vi "WSVCAP SHL Host LL Core.vi"(0 "Message In":string, 11 "error in":errorcluster, 12 "Log (T)":bool=TRUE, 13 "Function":T3) -> (3 "System":T1={"Settings"={"FPGA Resource Name"="", "I2C Slave Address"=20, "I2C Clock Rate (Hz)"=50000.0, "SPI Clock Rate (Hz)"=50000.0, "RFFE Slave Address"=20, "RFFE Clock Rate (Hz)"=50000.0, "Simulate FPGA"=TRUE, "C1 Cap DAC Default"=165, "C2 Cap DAC Default"=134, "C3 Cap DAC Default"=150}, "FPGA Resource"="", "Online"=FALSE, "I2C Wait Ticks"=0, "SPI Wait Ticks"=0, "RFFE Wait Ticks"=0} {"Settings"."C3 Cap DAC Default" format="0x%02x"; "Settings"."C2 Cap DAC Default" format="0x%02x"; "Settings"."C1 Cap DAC Default" format="0x%02x"; "Settings"."RFFE Clock Rate (Hz)" format="%.0f Hz"; "Settings"."RFFE Slave Address" format="0x%02x"; "Settings"."I2C Clock Rate (Hz)" format="%.0f Hz"; "Settings"."SPI Clock Rate (Hz)" format="%.0f Hz"; "Settings"."I2C Slave Address" format="0x%02x"}, 4 "Message Out":string, 15 "error out":errorcluster)   [LabVIEW 2012]
uses:
  Type Defs/WSVCAP SHL Function Enum.ctl
  Type Defs/WSVCAP SHL Core System Cluster.ctl
  Type Defs/WSVCAP SHL I2C Settings Cluster.ctl
  user.lib/Utilities/Type Defs/MISC IO Choice Enum.ctl
  Type Defs/WSVCAP SHL Top Level Control Operation Enum.ctl
  Type Defs/WSVCAP SHL Top Level Control Enum.ctl
  Type Defs/WSVCAP SHL Manager Operation Enum.ctl
  user.lib/Configuration Files/Type Defs/CFG File Operation Enum.ctl
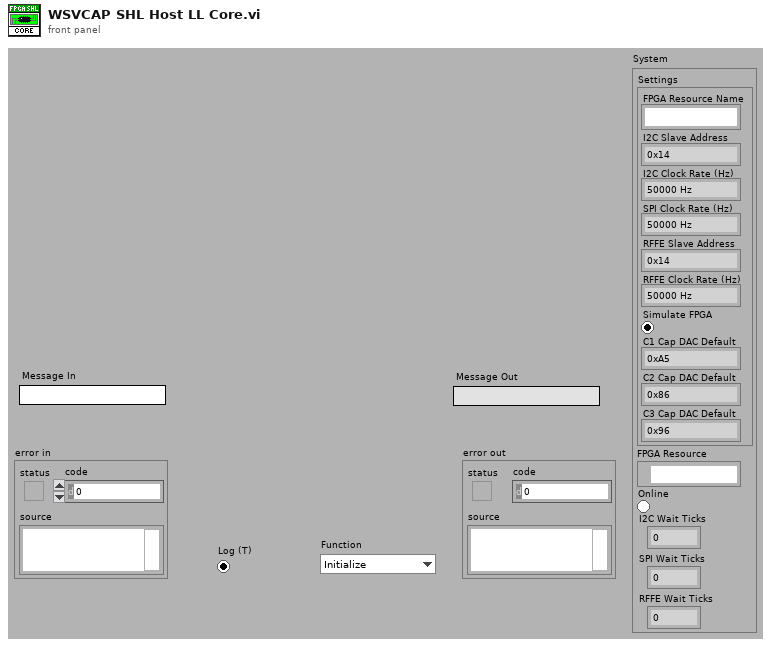
[diagram p1: front panel]
types:
  T1 = typedef "WSVCAP SHL Core System Cluster.ctl" = cluster{"Settings":T2, "FPGA Resource":tag, "Online":bool, "I2C Wait Ticks":u32, "SPI Wait Ticks":u32, "RFFE Wait Ticks":u32}
  T2 = typedef "WSVCAP SHL I2C Settings Cluster.ctl" = cluster{"FPGA Resource Name":string, "I2C Slave Address":u8, "I2C Clock Rate (Hz)":dbl, "SPI Clock Rate (Hz)":dbl, "RFFE Slave Address":u8, "RFFE Clock Rate (Hz)":dbl, "Simulate FPGA":bool, "C1 Cap DAC Default":u8, "C2 Cap DAC Default":u8, "C3 Cap DAC Default":u8}
  T3 = typedef "WSVCAP SHL Function Enum.ctl" = enum16{"Initialize", "Configure I2C", "Configure SPI", "Configure RFFE", "Write I2C", "Read I2C", "Write/Read SPI", "Start SPI Cycle", "Stop SPI Cycle", "Write RFFE", "Read RFFE", "Start RFFE Cycle", "Stop RFFE Cycle", "Get Status", "Close"}
  T4 = typedef "MISC IO Choice Enum.ctl" = enum16{"Read", "Write"}
  T5 = typedef "CFG File Operation Enum.ctl" = enum16{"Read", "Write", "Copy", "Edit"}
  T6 = typedef "WSVCAP SHL Manager Operation Enum.ctl" = enum16{"Initialize", "Close"}
  T7 = typedef "WSVCAP SHL Top Level Control Enum.ctl" = enum16{"Start", "Cmd", "Transaction", "Wait Ticks", "Socket Mask", "Slave Address", "Sub Address", "Bytes to Write", "Bytes to Read", "Write Data", "Write Flag", "Read Data", "Read Flag", "Ack Read", "Read Status Flag", "Ack Read Status", "Status", "Cycle Count", "Stop Cycle", "Exit"}
  T8 = typedef "WSVCAP SHL Top Level Control Operation Enum.ctl" = enum16{"Initialize", "Set Control", "Read Control", "Close"}
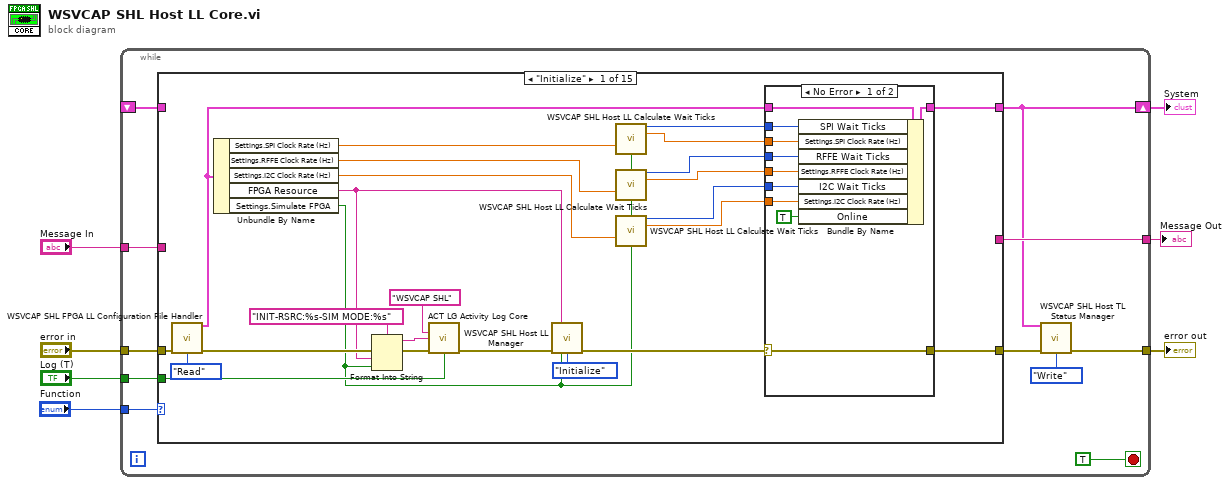
[diagram p0: block diagram]
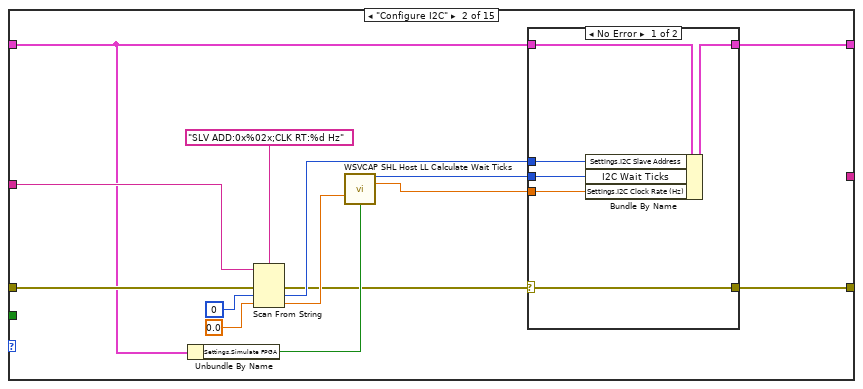
[diagram p3: hidden frame]
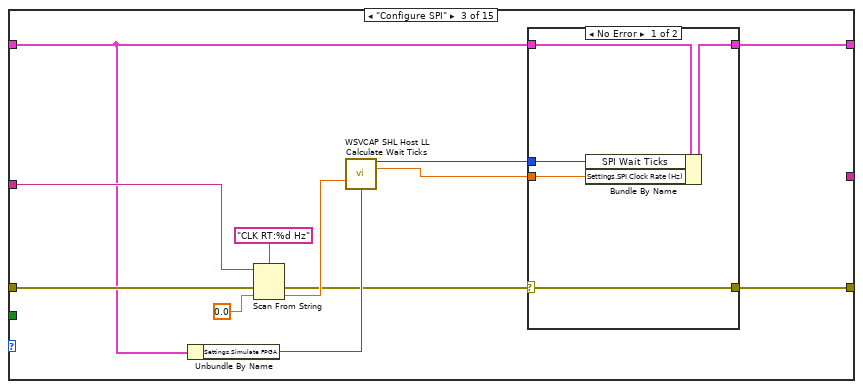
[diagram p5: hidden frame]
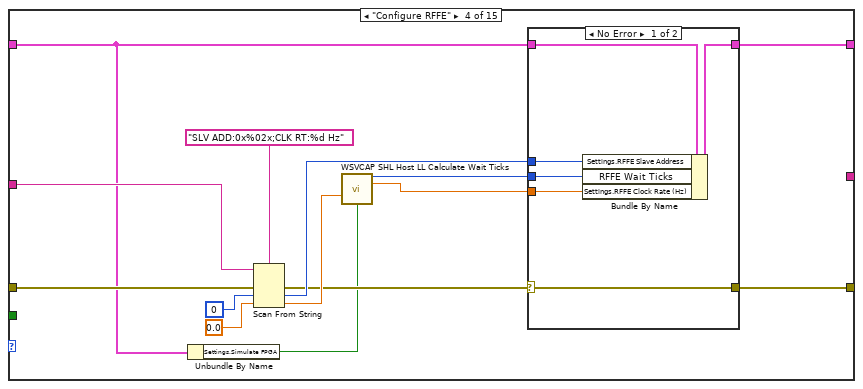
[diagram p7: hidden frame]
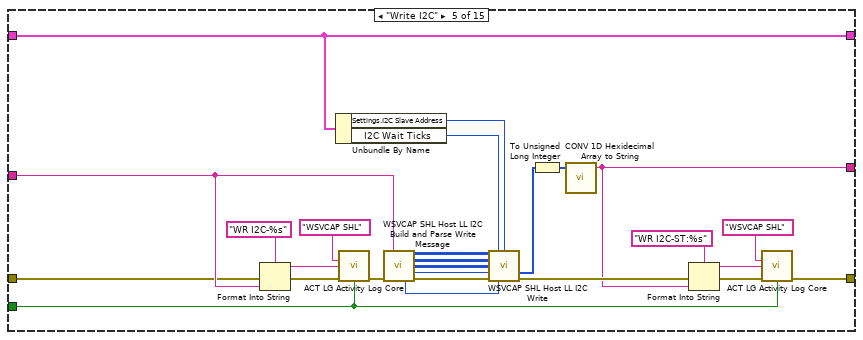
[diagram p9: hidden frame]
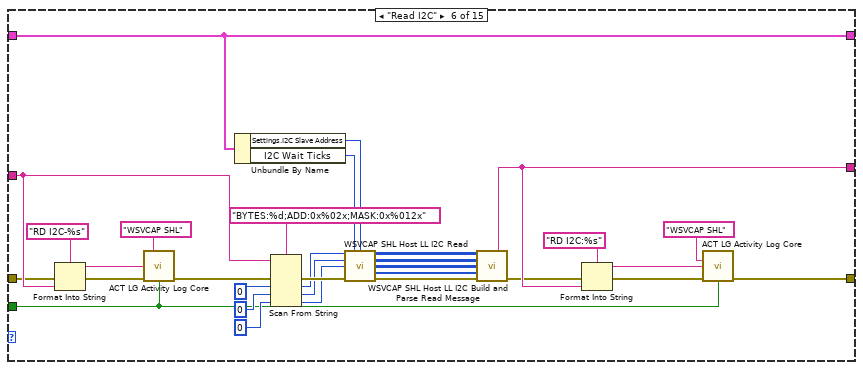
[diagram p10: hidden frame]
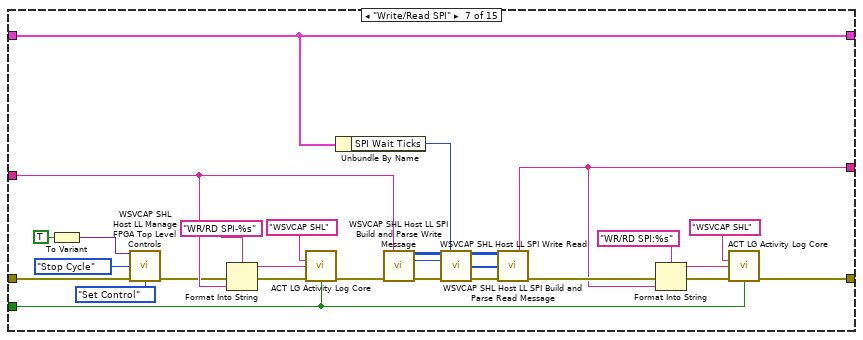
[diagram p11: hidden frame]
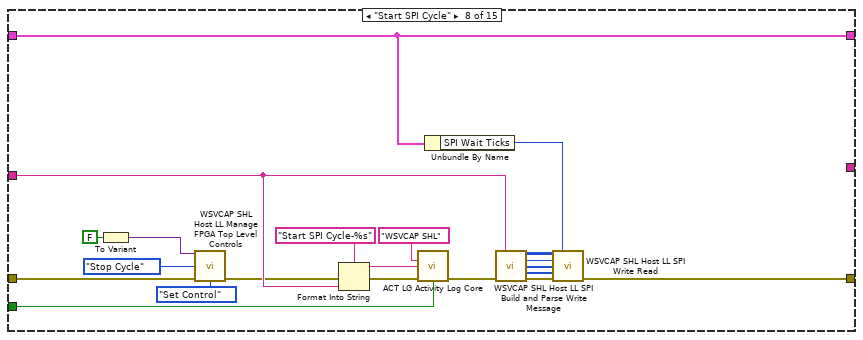
[diagram p12: hidden frame]
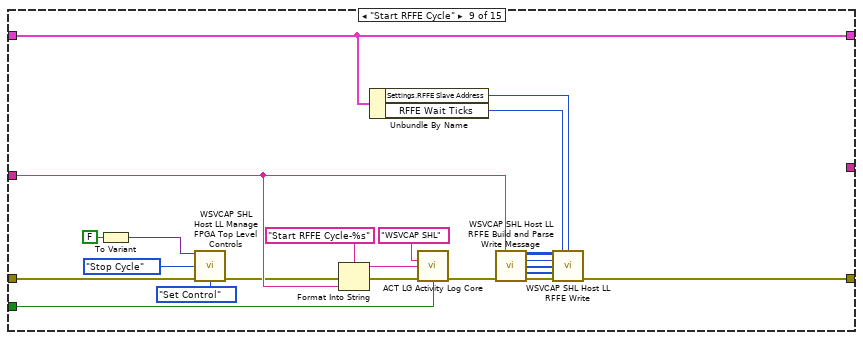
[diagram p13: hidden frame]
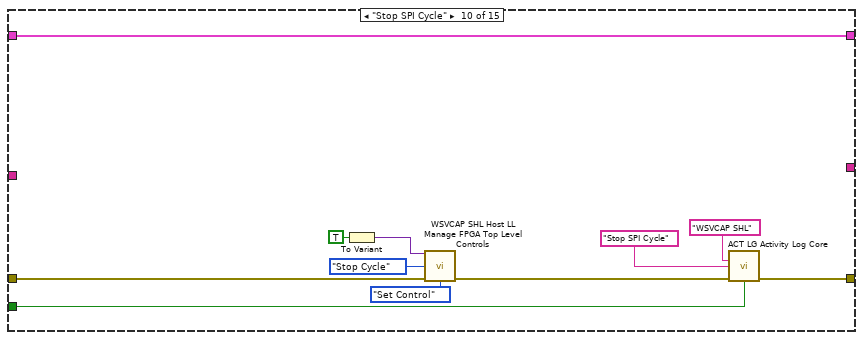
[diagram p14: hidden frame]
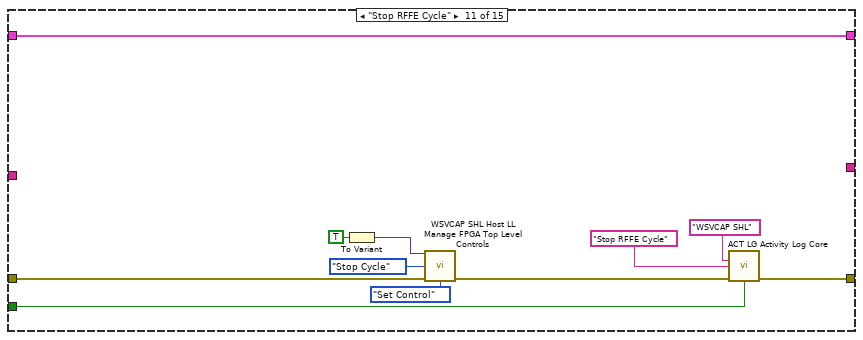
[diagram p15: hidden frame]
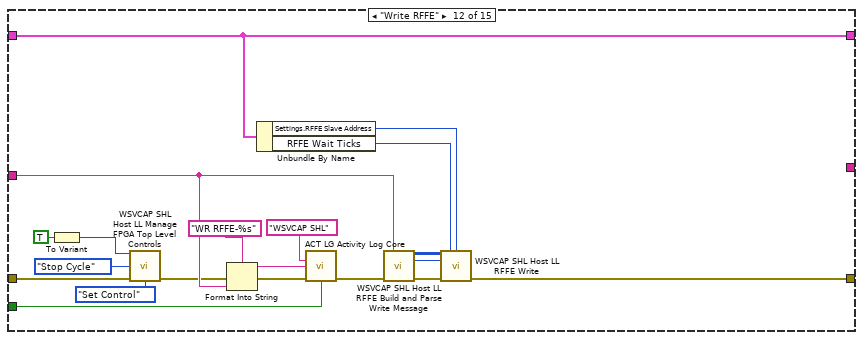
[diagram p16: hidden frame]
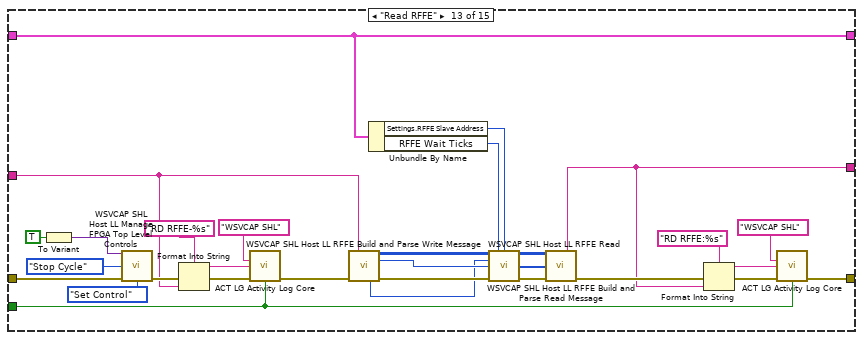
[diagram p17: hidden frame]
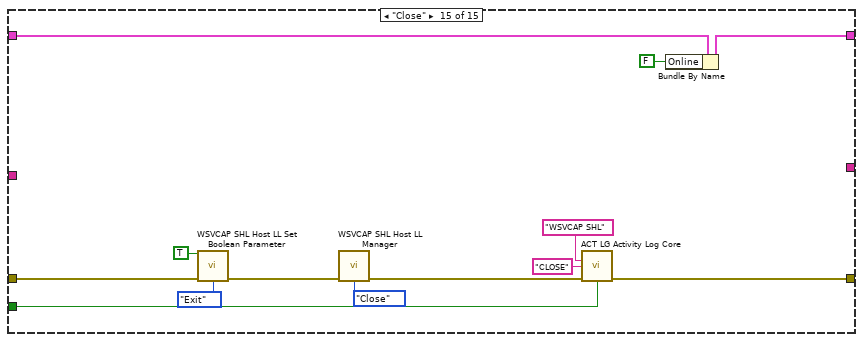
[diagram p19: hidden frame]
diagram:
  n1 = while {
    tunnel: "Function" -> [w17]
    tunnel: "error in" -> [w16]
    tunnel: "Message In" -> [w15]
    tunnel: [w11] -> w4
    shift-right: [w9] -> w3
    shift-left: _ -> [w14]
    tunnel: [w13] -> w2
    tunnel: "Log (T)" -> [w8]
    stop <- TRUE ("stop") stop-if-true
    n2 = case shown="\"Initialize\"" w17 {
      tunnel: w16 -> [w37 w67 w87 w108 w135 w156 w180 w207 w229 w248 w259 w275 w299 w319 w329]
      tunnel: w15 -> [_ w66 w86 w107 w136 w157 w186 w217 w239 _ _ w281 w292 _ _]
      tunnel: [w40 w68 w88 w109 w137 w153 w188 w215 w237 w255 w266 w270 w306 w319 w323] -> w12
      tunnel: [w41 w69 w89 w110 w123 w149 w177 w205 w227 w257 w268 w272 w297 w320 w332] -> w9
      tunnel: w14 -> [_ w62 w84 w103 w123 w149 w177 w205 w227 w257 w268 w272 w297 w320 w327]
      tunnel: [_ _ _ _ w127 w158 w187 _ _ _ _ _ w305 _ _] -> w13
      tunnel: w8 -> [w28 _ _ _ w124 w150 w185 w216 w238 w254 w265 w280 w304 _ w321]
      frame "Initialize" {
        n3 = call "WSVCAP SHL FPGA LL Configuration File Handler.vi"("Error In (no error)"=w37, "Operation"=CFG_File_Operation_Enum."Read") -> ("Object Cluster Out"=w42:T1, "Error Out"=w34:errorcluster)  [unwired: 11 in, 1 out]
        n4 = Unbundle By Name(w42) -> ("Settings.SPI Clock Rate (Hz)"=w22:dbl, "Settings.RFFE Clock Rate (Hz)"=w26:dbl, "Settings.I2C Clock Rate (Hz)"=w30:dbl, "FPGA Resource"=w31:tag, "Settings.Simulate FPGA"=w19:bool)
        n5 = Format Into String(format string="INIT-RSRC:%s-SIM MODE:%s", error in=w34, w31, w19) -> (resulting string=w35:string, error out=w33:errorcluster)  [unwired: 1 in]
        n6 = call "ACT LG Activity Log Core.vi"("Source"="WSVCAP SHL", "Log Line"=w35, "Error In (no error)"=w33, "Log (T)"=w28) -> ("Error Out"=w36:errorcluster)  [unwired: 10 in, 1 out]
        n7 = call "WSVCAP SHL Host LL Manager.vi"("FPGA Resource (Init Only)"=w31, "error in (no error)"=w36, "Simulate FPGA (Init Only)"=w19, "Operation"=WSVCAP_SHL_Manager_Operation_Enum."Initialize") -> ("error out"=w23:errorcluster)  [unwired: 11 in]
        n8 = call "WSVCAP SHL Host LL Calculate Wait Ticks.vi"("Clock Rate (Hz)"=w22, "Simulate FPGA"=w19) -> ("Wait Ticks"=w21:u32, "Actual Rate (Hz)"=w20:dbl)  [unwired: 12 in]
        n9 = call "WSVCAP SHL Host LL Calculate Wait Ticks.vi"("Clock Rate (Hz)"=w26, "Simulate FPGA"=w19) -> ("Wait Ticks"=w25:u32, "Actual Rate (Hz)"=w24:dbl)  [unwired: 12 in]
        n10 = call "WSVCAP SHL Host LL Calculate Wait Ticks.vi"("Clock Rate (Hz)"=w30, "Simulate FPGA"=w19) -> ("Wait Ticks"=w27:u32, "Actual Rate (Hz)"=w39:dbl)  [unwired: 12 in]
        n11 = case shown="No Error" w23 {
          selector: w23 -> [w51 w54]
          tunnel: w42 -> [w53 w55]
          tunnel: [w52 w55] -> w41
          tunnel: [w51 w54] -> w40
          tunnel: w39 -> [w50 _]
          tunnel: w27 -> [w48 _]
          tunnel: w25 -> [w47 _]
          tunnel: w24 -> [w46 _]
          tunnel: w21 -> [w45 _]
          tunnel: w20 -> [w44 _]
          frame No Error {
            n12 = Bundle By Name(cluster=w53, "SPI Wait Ticks"=w45, "Settings.SPI Clock Rate (Hz)"=w44, "RFFE Wait Ticks"=w47, "Settings.RFFE Clock Rate (Hz)"=w46, "I2C Wait Ticks"=w48, "Settings.I2C Clock Rate (Hz)"=w50, "Online"=TRUE) -> (w52:T1)
          }
          frame Error {
          }
        }
      }
      frame "Configure I2C" {
        n13 = Unbundle By Name(w62) -> ("Settings.Simulate FPGA"=w61:bool)
        n14 = Scan From String(format string="SLV ADD:0x%02x;CLK RT:%d Hz", input string=w66, error in=w67, default 1=u8 0 ("I2C_Slave Address"), default 2=0.0 ("Clock Rate (Hz)")) -> (error out=w56:errorcluster, output 1=w63:u8, output 2=w59:dbl)  [unwired: 1 in, 2 out]
        n15 = call "WSVCAP SHL Host LL Calculate Wait Ticks.vi"("Clock Rate (Hz)"=w59, "Simulate FPGA"=w61) -> ("Wait Ticks"=w57:u32, "Actual Rate (Hz)"=w58:dbl)  [unwired: 12 in]
        n16 = case shown="No Error" w56 {
          selector: w56 -> [w73 w76]
          tunnel: w62 -> [w75 w77]
          tunnel: [w74 w77] -> w69
          tunnel: [w73 w76] -> w68
          tunnel: w63 -> [w72 _]
          tunnel: w58 -> [w71 _]
          tunnel: w57 -> [w70 _]
          frame No Error {
            n17 = Bundle By Name(cluster=w75, "Settings.I2C Slave Address"=w72, "I2C Wait Ticks"=w70, "Settings.I2C Clock Rate (Hz)"=w71) -> (w74:T1)
          }
          frame Error {
          }
        }
      }
      frame "Configure SPI" {
        n18 = Unbundle By Name(w84) -> ("Settings.Simulate FPGA"=w79:bool)
        n19 = Scan From String(format string="CLK RT:%d Hz", input string=w86, error in=w87, default 1=0.0 ("Clock Rate (Hz)")) -> (error out=w78:errorcluster, output 1=w82:dbl)  [unwired: 1 in, 2 out]
        n20 = call "WSVCAP SHL Host LL Calculate Wait Ticks.vi"("Clock Rate (Hz)"=w82, "Simulate FPGA"=w79) -> ("Wait Ticks"=w81:u32, "Actual Rate (Hz)"=w80:dbl)  [unwired: 12 in]
        n21 = case shown="No Error" w78 {
          selector: w78 -> [w92 w95]
          tunnel: w84 -> [w94 w96]
          tunnel: [w93 w96] -> w89
          tunnel: [w92 w95] -> w88
          tunnel: w80 -> [w91 _]
          tunnel: w81 -> [w90 _]
          frame No Error {
            n22 = Bundle By Name(cluster=w94, "SPI Wait Ticks"=w90, "Settings.SPI Clock Rate (Hz)"=w91) -> (w93:T1)
          }
          frame Error {
          }
        }
      }
      frame "Configure RFFE" {
        n23 = Unbundle By Name(w103) -> ("Settings.Simulate FPGA"=w97:bool)
        n24 = Scan From String(format string="SLV ADD:0x%02x;CLK RT:%d Hz", input string=w107, error in=w108, default 1=u8 0 ("I2C_Slave Address"), default 2=0.0 ("Clock Rate (Hz)")) -> (error out=w98:errorcluster, output 1=w104:u8, output 2=w101:dbl)  [unwired: 1 in, 2 out]
        n25 = call "WSVCAP SHL Host LL Calculate Wait Ticks.vi"("Clock Rate (Hz)"=w101, "Simulate FPGA"=w97) -> ("Wait Ticks"=w100:u32, "Actual Rate (Hz)"=w99:dbl)  [unwired: 12 in]
        n26 = case shown="No Error" w98 {
          selector: w98 -> [w114 w117]
          tunnel: w103 -> [w116 w118]
          tunnel: [w115 w118] -> w110
          tunnel: [w114 w117] -> w109
          tunnel: w104 -> [w113 _]
          tunnel: w99 -> [w112 _]
          tunnel: w100 -> [w111 _]
          frame No Error {
            n27 = Bundle By Name(cluster=w116, "Settings.RFFE Slave Address"=w113, "RFFE Wait Ticks"=w111, "Settings.RFFE Clock Rate (Hz)"=w112) -> (w115:T1)
          }
          frame Error {
          }
        }
      }
      frame "Write I2C" {
        n28 = Format Into String(format string="WR I2C-%s", error in=w135, w136) -> (resulting string=w132:string, error out=w134:errorcluster)  [unwired: 1 in]
        n29 = Unbundle By Name(w123) -> ("Settings.I2C Slave Address"=w119:u8, "I2C Wait Ticks"=w122:u32)
        n30 = call "ACT LG Activity Log Core.vi"("Source"="WSVCAP SHL", "Log Line"=w132, "Error In (no error)"=w134, "Log (T)"=w124) -> ("Error Out"=w139:errorcluster)  [unwired: 10 in, 1 out]
        n31 = call "WSVCAP SHL Host LL I2C Build and Parse Write Message.vi"("Message In"=w136, "error in"=w139) -> ("C1 Write Data Out [DUT Ordered]"=w143:u8[][], "C2 Write Data Out [DUT Ordered]"=w141:u8[][], "C3 Write Data Out [DUT Ordered]"=w121:u8[][], "Socket Mask [U64] Out"=w142:u64, "Sub Address Out"=w120:u8, "error out"=w144:errorcluster)  [unwired: 7 in, 1 out]
        n32 = call "WSVCAP SHL Host LL I2C Write.vi"("C1 Data Out [DUT Ordered]"=w143, "Wait Ticks"=w122, "Slave Address"=w119, "C2 Data Out [DUT Ordered]"=w141, "C3 Data Out [DUT Ordered]"=w121, "Socket Mask [U64]"=w142, "error in"=w144, "Sub Address"=w120) -> ("Status"=w129:u8[], "error out"=w131:errorcluster)  [unwired: 6 in]
        n33 = To Unsigned Long Integer(number=w129) -> (unsigned 32bit integer=w128:u32[])
        n34 = call "CONV 1D Hexidecimal Array to String.vi"("1-D Hexidecimal"=w128) -> ("String"=w127:string)  [unwired: 8 in]
        n35 = Format Into String(format string="WR I2C-ST:%s", error in=w131, w127) -> (resulting string=w125:string, error out=w130:errorcluster)  [unwired: 1 in]
        n36 = call "ACT LG Activity Log Core.vi"("Source"="WSVCAP SHL", "Log Line"=w125, "Error In (no error)"=w130, "Log (T)"=w124) -> ("Error Out"=w137:errorcluster)  [unwired: 10 in, 1 out]
      }
      frame "Read I2C" {
        n37 = Format Into String(format string="RD I2C-%s", error in=w156, w157) -> (resulting string=w162:string, error out=w164:errorcluster)  [unwired: 1 in]
        n38 = call "ACT LG Activity Log Core.vi"("Source"="WSVCAP SHL", "Log Line"=w162, "Error In (no error)"=w164, "Log (T)"=w150) -> ("Error Out"=w155:errorcluster)  [unwired: 10 in, 1 out]
        n39 = Unbundle By Name(w149) -> ("Settings.I2C Slave Address"=w145:u8, "I2C Wait Ticks"=w148:u32)
        n40 = Scan From String(format string="BYTES:%d;ADD:0x%02x;MASK:0x%012x", input string=w157, error in=w155, default 1=u8 0 ("Bytes to Read"), default 2=u8 0 ("Sub Address [U8]"), default 3=u64 0 ("Socket Mask [U32]")) -> (error out=w175:errorcluster, output 1=w171:u8, output 2=w169:u8, output 3=w170:u64)  [unwired: 1 in, 2 out]
        n41 = call "WSVCAP SHL Host LL I2C Read.vi"("Bytes to Read"=w171, "Wait Ticks"=w148, "Slave Address"=w145, "Sub Address [U8]"=w169, "Socket Mask [U64]"=w170, "error in"=w175) -> ("C1:1-16 Read Data [DUT Ordered]"=w167:u8[][], "C2:1-16 Read Data [DUT Ordered]"=w166:u8[][], "C3:1-16 Read Data [DUT Ordered]"=w147:u8[][], "Status"=w146:u8[], "error out"=w168:errorcluster)  [unwired: 5 in]
        n42 = call "WSVCAP SHL Host LL I2C Build and Parse Read Message.vi"("C1 Write Data In"=w167, "C2 Write Data"=w166, "C3 Write Data"=w147, "Status In"=w146, "error in"=w168) -> ("Message Out"=w158:string, "error out"=w154:errorcluster)  [unwired: 5 in, 4 out]
        n43 = Format Into String(format string="RD I2C:%s", error in=w154, w158) -> (resulting string=w159:string, error out=w161:errorcluster)  [unwired: 1 in]
        n44 = call "ACT LG Activity Log Core.vi"("Source"="WSVCAP SHL", "Log Line"=w159, "Error In (no error)"=w161, "Log (T)"=w150) -> ("Error Out"=w153:errorcluster)  [unwired: 10 in, 1 out]
      }
      frame "Write/Read SPI" {
        n45 = To Variant(anything=TRUE ("Cycle (F:Write/Read - T:Write Only - No Read)")) -> (Variant=w182:variant)
        n46 = call "WSVCAP SHL Host LL Manage FPGA Top Level Controls.vi"("Value In"=w182, "FPGA Top Level Control"=WSVCAP_SHL_Top_Level_Control_Enum."Stop Cycle", "error in (no error)"=w180, "Operation"=WSVCAP_SHL_Top_Level_Control_Operation_Enum."Set Control") -> ("error out"=w179:errorcluster)  [unwired: 10 in, 1 out]
        n47 = Format Into String(format string="WR/RD SPI-%s", error in=w179, w186) -> (resulting string=w194:string, error out=w196:errorcluster)  [unwired: 1 in]
        n48 = call "ACT LG Activity Log Core.vi"("Source"="WSVCAP SHL", "Log Line"=w194, "Error In (no error)"=w196, "Log (T)"=w185) -> ("Error Out"=w190:errorcluster)  [unwired: 10 in, 1 out]
        n49 = Unbundle By Name(w177) -> ("SPI Wait Ticks"=w176:u32)
        n50 = call "WSVCAP SHL Host LL SPI Build and Parse Write Message.vi"("Message In"=w186, "error in"=w190) -> ("Write Data Out [DUT Ordered]"=w202:u8[][], "Socket Mask [U16] Out"=w178:u16, "error out"=w203:errorcluster)  [unwired: 8 in, 3 out]
        n51 = call "WSVCAP SHL Host LL SPI Write Read.vi"("SPI Data [DUT Ordered]"=w202, "Wait Ticks"=w176, "Socket Mask"=w178, "error in"=w203) -> ("SPI Read Data [DUT Ordered]"=w200:u8[][], "Status"=w199:u8[], "error out"=w201:errorcluster)  [unwired: 9 in]
        n52 = call "WSVCAP SHL Host LL SPI Build and Parse Read Message.vi"("Write Data In"=w200, "Status In"=w199, "error in"=w201) -> ("Message Out"=w187:string, "error out"=w189:errorcluster)  [unwired: 9 in, 2 out]
        n53 = Format Into String(format string="WR/RD SPI:%s", error in=w189, w187) -> (resulting string=w191:string, error out=w193:errorcluster)  [unwired: 1 in]
        n54 = call "ACT LG Activity Log Core.vi"("Source"="WSVCAP SHL", "Log Line"=w191, "Error In (no error)"=w193, "Log (T)"=w185) -> ("Error Out"=w188:errorcluster)  [unwired: 10 in, 1 out]
      }
      frame "Start SPI Cycle" {
        n55 = To Variant(anything=FALSE ("Cycle (F:Write/Read - T:Write Only - No Read)")) -> (Variant=w212:variant)
        n56 = call "WSVCAP SHL Host LL Manage FPGA Top Level Controls.vi"("Value In"=w212, "FPGA Top Level Control"=WSVCAP_SHL_Top_Level_Control_Enum."Stop Cycle", "error in (no error)"=w207, "Operation"=WSVCAP_SHL_Top_Level_Control_Operation_Enum."Set Control") -> ("error out"=w206:errorcluster)  [unwired: 10 in, 1 out]
        n57 = Format Into String(format string="Start SPI Cycle-%s", error in=w206, w217) -> (resulting string=w219:string, error out=w221:errorcluster)  [unwired: 1 in]
        n58 = call "ACT LG Activity Log Core.vi"("Source"="WSVCAP SHL", "Log Line"=w219, "Error In (no error)"=w221, "Log (T)"=w216) -> ("Error Out"=w218:errorcluster)  [unwired: 10 in, 1 out]
        n59 = Unbundle By Name(w205) -> ("SPI Wait Ticks"=w204:u32)
        n60 = call "WSVCAP SHL Host LL SPI Build and Parse Write Message.vi"("Message In"=w217, "error in"=w218) -> ("Write Data Out [DUT Ordered]"=w223:u8[][], "Socket Mask [U16] Out"=w210:u16, "Cycle CMD Lengths Out (bits)"=w209:u8[], "Cycle CMD Delay Out (ticks)"=w208:u32[], "error out"=w224:errorcluster)  [unwired: 8 in, 1 out]
        n61 = call "WSVCAP SHL Host LL SPI Write Read.vi"("SPI Data [DUT Ordered]"=w223, "Wait Ticks"=w204, "Socket Mask"=w210, "Cycle CMD Lengths Out (bits)"=w209, "Cycle CMD Delay Out (ticks)"=w208, "error in"=w224) -> ("error out"=w215:errorcluster)  [unwired: 7 in, 2 out]
      }
      frame "Start RFFE Cycle" {
        n62 = To Variant(anything=FALSE ("Cycle (F:Write/Read - T:Write Only - No Read)")) -> (Variant=w234:variant)
        n63 = call "WSVCAP SHL Host LL Manage FPGA Top Level Controls.vi"("Value In"=w234, "FPGA Top Level Control"=WSVCAP_SHL_Top_Level_Control_Enum."Stop Cycle", "error in (no error)"=w229, "Operation"=WSVCAP_SHL_Top_Level_Control_Operation_Enum."Set Control") -> ("error out"=w228:errorcluster)  [unwired: 10 in, 1 out]
        n64 = Format Into String(format string="Start RFFE Cycle-%s", error in=w228, w239) -> (resulting string=w241:string, error out=w243:errorcluster)  [unwired: 1 in]
        n65 = Unbundle By Name(w227) -> ("Settings.RFFE Slave Address"=w225:u8, "RFFE Wait Ticks"=w226:u32)
        n66 = call "ACT LG Activity Log Core.vi"("Source"="WSVCAP SHL", "Log Line"=w241, "Error In (no error)"=w243, "Log (T)"=w238) -> ("Error Out"=w240:errorcluster)  [unwired: 10 in, 1 out]
        n67 = call "WSVCAP SHL Host LL RFFE Build and Parse Write Message.vi"("Message In"=w239, "error in"=w240) -> ("Write Data Out [DUT Ordered]"=w245:u8[][], "Socket Mask [U16] Out"=w232:u16, "Cycle CMD Lengths Out (bits)"=w231:u8[], "Cycle CMD Delay Out (ticks)"=w230:u32[], "error out"=w246:errorcluster)  [unwired: 7 in, 2 out]
        n68 = call "WSVCAP SHL Host LL RFFE Write.vi"("RTFFE Data [DUT Ordered]"=w245, "Wait Ticks"=w226, "Slave Address"=w225, "Socket Mask"=w232, "Cycle CMD Lengths Out (bits)"=w231, "Cycle CMD Delay Out (ticks)"=w230, "error in"=w246) -> ("error out"=w237:errorcluster)  [unwired: 7 in, 1 out]
      }
      frame "Stop SPI Cycle" {
        n69 = To Variant(anything=TRUE ("Cycle (F:Write/Read - T:Write Only - No Read)")) -> (Variant=w250:variant)
        n70 = call "WSVCAP SHL Host LL Manage FPGA Top Level Controls.vi"("Value In"=w250, "FPGA Top Level Control"=WSVCAP_SHL_Top_Level_Control_Enum."Stop Cycle", "error in (no error)"=w248, "Operation"=WSVCAP_SHL_Top_Level_Control_Operation_Enum."Set Control") -> ("error out"=w247:errorcluster)  [unwired: 10 in, 1 out]
        n71 = call "ACT LG Activity Log Core.vi"("Source"="WSVCAP SHL", "Log Line"="Stop SPI Cycle" ("format string"), "Error In (no error)"=w247, "Log (T)"=w254) -> ("Error Out"=w255:errorcluster)  [unwired: 10 in, 1 out]
      }
      frame "Stop RFFE Cycle" {
        n72 = To Variant(anything=TRUE ("Cycle (F:Write/Read - T:Write Only - No Read)")) -> (Variant=w261:variant)
        n73 = call "WSVCAP SHL Host LL Manage FPGA Top Level Controls.vi"("Value In"=w261, "FPGA Top Level Control"=WSVCAP_SHL_Top_Level_Control_Enum."Stop Cycle", "error in (no error)"=w259, "Operation"=WSVCAP_SHL_Top_Level_Control_Operation_Enum."Set Control") -> ("error out"=w258:errorcluster)  [unwired: 10 in, 1 out]
        n74 = call "ACT LG Activity Log Core.vi"("Source"="WSVCAP SHL", "Log Line"="Stop RFFE Cycle" ("format string"), "Error In (no error)"=w258, "Log (T)"=w265) -> ("Error Out"=w266:errorcluster)  [unwired: 10 in, 1 out]
      }
      frame "Write RFFE" {
        n75 = To Variant(anything=TRUE ("Cycle (F:Write/Read - T:Write Only - No Read)")) -> (Variant=w277:variant)
        n76 = call "WSVCAP SHL Host LL Manage FPGA Top Level Controls.vi"("Value In"=w277, "FPGA Top Level Control"=WSVCAP_SHL_Top_Level_Control_Enum."Stop Cycle", "error in (no error)"=w275, "Operation"=WSVCAP_SHL_Top_Level_Control_Operation_Enum."Set Control") -> ("error out"=w274:errorcluster)  [unwired: 10 in, 1 out]
        n77 = Format Into String(format string="WR RFFE-%s", error in=w274, w281) -> (resulting string=w283:string, error out=w285:errorcluster)  [unwired: 1 in]
        n78 = Unbundle By Name(w272) -> ("Settings.RFFE Slave Address"=w269:u8, "RFFE Wait Ticks"=w271:u32)
        n79 = call "ACT LG Activity Log Core.vi"("Source"="WSVCAP SHL", "Log Line"=w283, "Error In (no error)"=w285, "Log (T)"=w280) -> ("Error Out"=w282:errorcluster)  [unwired: 10 in, 1 out]
        n80 = call "WSVCAP SHL Host LL RFFE Build and Parse Write Message.vi"("Message In"=w281, "error in"=w282) -> ("Write Data Out [DUT Ordered]"=w287:u8[][], "Socket Mask [U16] Out"=w273:u16, "error out"=w288:errorcluster)  [unwired: 7 in, 4 out]
        n81 = call "WSVCAP SHL Host LL RFFE Write.vi"("RTFFE Data [DUT Ordered]"=w287, "Wait Ticks"=w271, "Slave Address"=w269, "Socket Mask"=w273, "error in"=w288) -> ("error out"=w270:errorcluster)  [unwired: 9 in, 1 out]
      }
      frame "Read RFFE" {
        n82 = To Variant(anything=TRUE ("Cycle (F:Write/Read - T:Write Only - No Read)")) -> (Variant=w301:variant)
        n83 = call "WSVCAP SHL Host LL Manage FPGA Top Level Controls.vi"("Value In"=w301, "FPGA Top Level Control"=WSVCAP_SHL_Top_Level_Control_Enum."Stop Cycle", "error in (no error)"=w299, "Operation"=WSVCAP_SHL_Top_Level_Control_Operation_Enum."Set Control") -> ("error out"=w298:errorcluster)  [unwired: 10 in, 1 out]
        n84 = Format Into String(format string="RD RFFE-%s", error in=w298, w292) -> (resulting string=w311:string, error out=w313:errorcluster)  [unwired: 1 in]
        n85 = call "ACT LG Activity Log Core.vi"("Source"="WSVCAP SHL", "Log Line"=w311, "Error In (no error)"=w313, "Log (T)"=w304) -> ("Error Out"=w294:errorcluster)  [unwired: 10 in, 1 out]
        n86 = call "WSVCAP SHL Host LL RFFE Build and Parse Write Message.vi"("Message In"=w292, "error in"=w294) -> ("Write Data Out [DUT Ordered]"=w291:u8[][], "Socket Mask [U16] Out"=w290:u16, "Byte Count"=w289:u8, "error out"=w293:errorcluster)  [unwired: 7 in, 3 out]
        n87 = Unbundle By Name(w297) -> ("Settings.RFFE Slave Address"=w295:u8, "RFFE Wait Ticks"=w296:u32)
        n88 = call "WSVCAP SHL Host LL RFFE Read.vi"("RFFE Data [DUT Ordered]"=w291, "Wait Ticks"=w296, "Slave Address"=w295, "Bytes to Read"=w289, "Socket Mask [U16]"=w290, "error in"=w293) -> ("RFFE Read Data [DUT Ordered]"=w317:u8[][], "Status"=w316:u8[], "error out"=w318:errorcluster)  [unwired: 7 in]
        n89 = call "WSVCAP SHL Host LL RFFE Build and Parse Read Message.vi"("Write Data In"=w317, "Status In"=w316, "error in"=w318) -> ("Message Out"=w305:string, "error out"=w307:errorcluster)  [unwired: 9 in, 2 out]
        n90 = Format Into String(format string="RD RFFE:%s", error in=w307, w305) -> (resulting string=w308:string, error out=w310:errorcluster)  [unwired: 1 in]
        n91 = call "ACT LG Activity Log Core.vi"("Source"="WSVCAP SHL", "Log Line"=w308, "Error In (no error)"=w310, "Log (T)"=w304) -> ("Error Out"=w306:errorcluster)  [unwired: 10 in, 1 out]
      }
      frame "Get Status" {
      }
      frame "Close" {
        n92 = call "WSVCAP SHL Host LL Set Boolean Parameter.vi"("Boolean In"=TRUE ("Start"), "error in (no error)"=w329, "FPGA Top Level Control"=WSVCAP_SHL_Top_Level_Control_Enum."Exit") -> ("error out"=w328:errorcluster)  [unwired: 12 in]
        n93 = call "WSVCAP SHL Host LL Manager.vi"("error in (no error)"=w328, "Operation"=WSVCAP_SHL_Manager_Operation_Enum."Close") -> ("error out"=w324:errorcluster)  [unwired: 13 in]
        n94 = call "ACT LG Activity Log Core.vi"("Source"="WSVCAP SHL", "Log Line"="CLOSE", "Error In (no error)"=w324, "Log (T)"=w321) -> ("Error Out"=w323:errorcluster)  [unwired: 10 in, 1 out]
        n95 = Bundle By Name(cluster=w327, "Online"=FALSE) -> (w332:T1)
      }
    }
    n96 = call "WSVCAP SHL Host TL Status Manager.vi"("System In"=w9, "error in"=w12, "Operation (Read)"=MISC_IO_Choice_Enum."Write") -> ("error out"=w11:errorcluster)  [unwired: 11 in, 1 out]
  }
  "error out" <- w4
  "Message Out" <- w2
  "System" <- w3
